vi "Choose Drive Command.vi"() -> (0 "Current Drive Command":T1)   [LabVIEW 2019]
uses:
  .Team Code/Robot Global Data.vi
  Drive Command Typedef.ctl
  Drive Mode Typedef.ctl
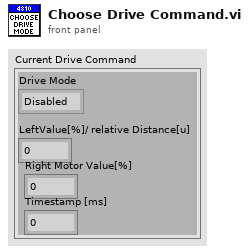
[diagram p1: front panel]
types:
  T1 = typedef "Drive Command Typedef.ctl" = cluster{"Drive Mode":T2, "LeftValue[%]/ relative Distance[u]":dbl, "Right Motor Value[%]":dbl, "Timestamp [ms]":dbl}
  T2 = typedef "Drive Mode Typedef.ctl" = enum16{"Disabled", "Auto-align", "Drive Distance", "Turn to angle", "Driver"}
  T3 = typedef "WPI_DriverStationRobotMode2.ctl" = enum16{"Autonomous Disabled", "Autonomous Enabled", "Teleop Disabled", "Teleop Enabled", "Disconnected", "Finish", "Test Disabled", "Test Enabled", "Emergency Stopped"}
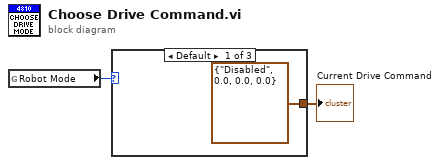
[diagram p0: block diagram]
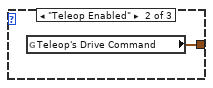
[diagram p2: hidden frame]
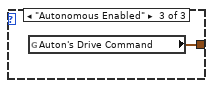
[diagram p3: hidden frame]
diagram:
  n1 = global read "Robot Global Data.vi" "Robot Mode"() -> (w2:T3)
  n2 = case shown="Default" w2 {
    tunnel: [T1 {"Drive Mode"=enum."Disabled", "LeftValue[%]/ relative Distance[u]"=0.0, "Right Motor Value[%]"=0.0, "Timestamp [ms]"=0.0} ("Drive Command") w4 w5] -> w1
    frame Default {
    }
    frame "Teleop Enabled" {
      n3 = global read "Robot Global Data.vi" "Teleop's Drive Command"() -> (w4:T1)
    }
    frame "Autonomous Enabled" {
      n4 = global read "Robot Global Data.vi" "Auton's Drive Command"() -> (w5:T1)
    }
  }
  "Current Drive Command" <- w1
